vi "DIFF_DRIVE_GLOBALS.vi"() -> ()   [LabVIEW 2023]
panel:
  out "Wheel Diameter IN":dbl
  out "Gear Ratio":dbl
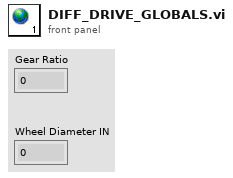
[diagram p1: front panel]
diagram:
